vi "AnalyseNISTvsFlukeResults.vi"(8 "error in (no error)":errorcluster, 10 "AllData In":T4 {"FlukeData"."DataAnalysisArray"."TimeStamp" format="%^<%.3X\n%x>T"; "FlukeData"."ModelDataArray"."FREQUENCY" format="%#_6f"; "FlukeData"."ModelDataArray"."TimeStamp" format="%^<%.3X\n%x>T"; "FlukeData"."PMUDataArray"."FREQUENCY" format="%#_6f"; "FlukeData"."PMUDataArray"."TimeStamp" format="%^<%.3X\n%x>T"; "NISTData"."DataAnlysisArray"."TimeStamp" format="%^<%.3X\n%x>T"; "NISTData"."DUTDataArray"."Time Stamp" format="%^<%.3X\n%x>T"; "NISTData"."NIDataArray"."Time Stamp" format="%^<%.3X\n%x>T"}, 11 "NISTResults":T3 {"Time Stamp" format="%^<%.3X\n%x>T"}) -> (0 "error out":errorcluster, 3 "Resultarray":T1[](array[typedef]) {"Time Stamp" format="%^<%.3X\n%x>T"})   [LabVIEW 2014]
uses:
  typedefs/Alldata.ctl
  typedefs/NISTData.ctl
  typedefs/NIDataArray.ctl
  typedefs/NIData.ctl
  typedefs/PhasorRectangular.ctl
  typedefs/DUTData.ctl
  typedefs/NICalcAnalysis.ctl
  typedefs/CalcPhasorError.ctl
  typedefs/PlotDataArrays.ctl
  typedefs/PmuRawDataCluster.ctl
  typedefs/CalcAnalysis.ctl
  typedefs/ResultArray.ctl
  typedefs/Result.ctl
  typedefs/TVE_Fe_RFE.ctl
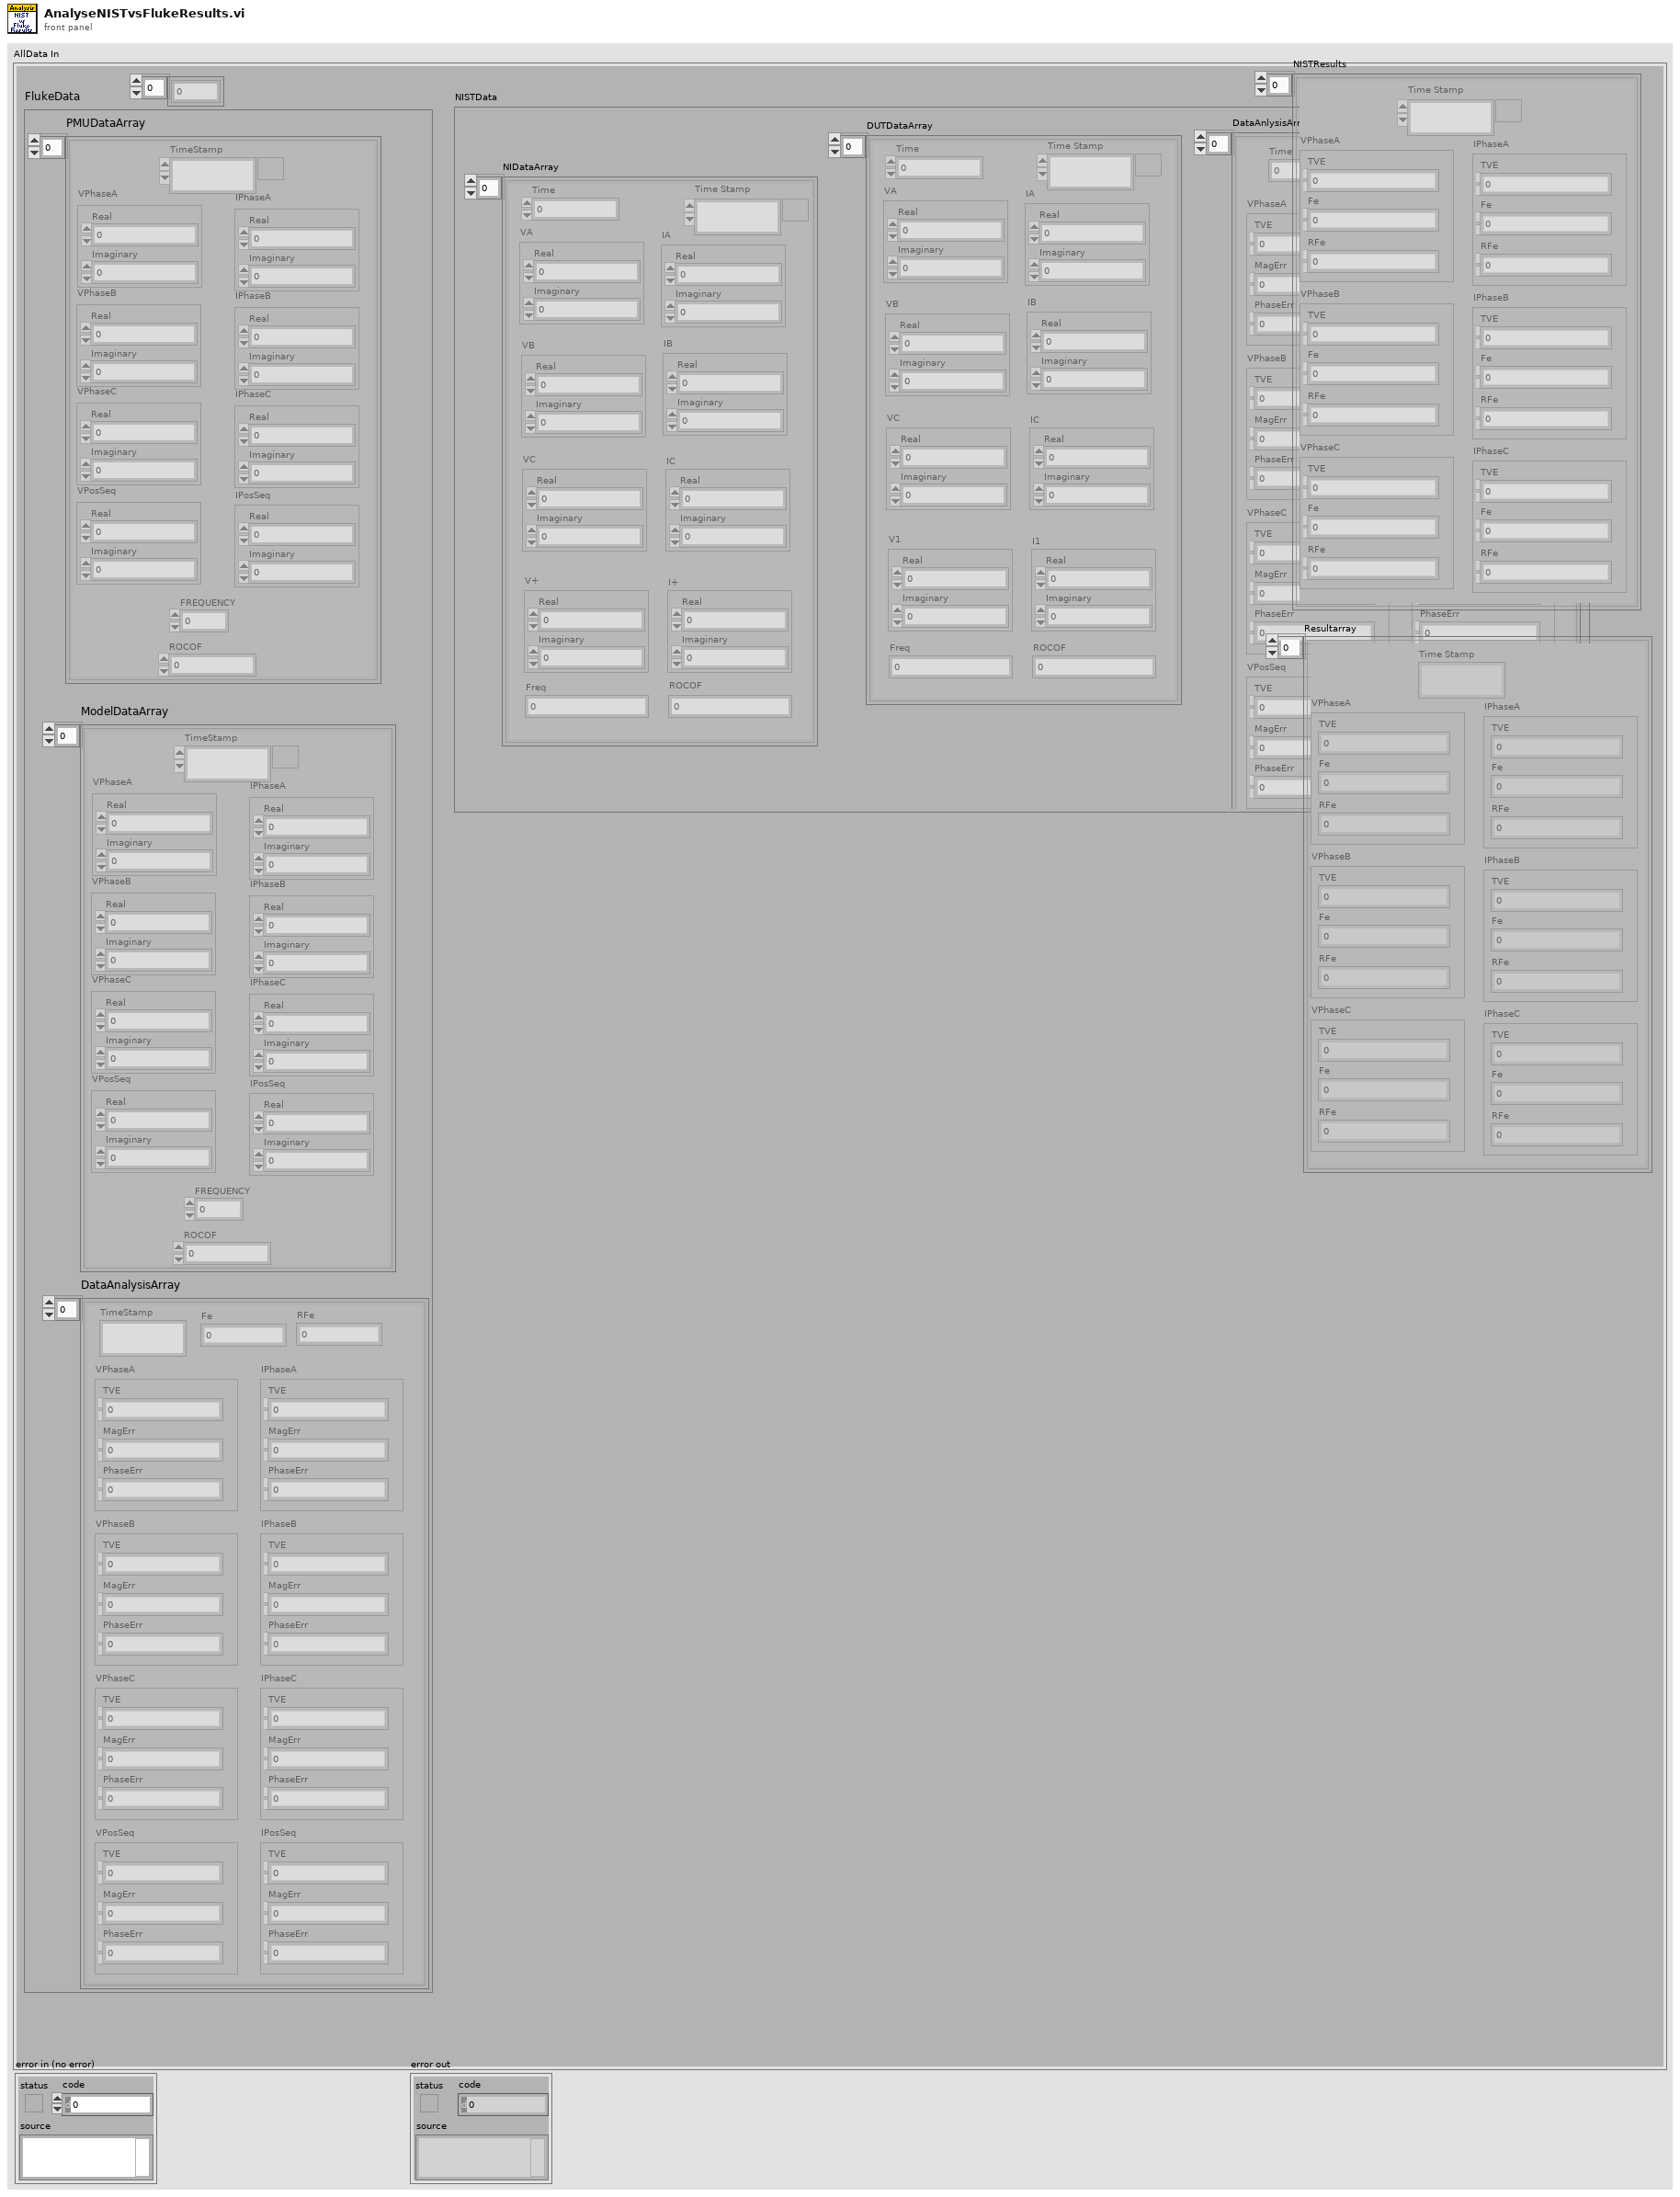
[diagram p1: front panel]
types:
  T1 = typedef "Result.ctl" = cluster{"Time Stamp":timestamp, "VPhaseA":T2, "VPhaseB":T2, "VPhaseC":T2, "IPhaseA":T2, "IPhaseB":T2, "IPhaseC":T2}
  T2 = typedef "TVE_Fe_RFE.ctl" = cluster{"TVE":dbl, "Fe":dbl, "RFe":dbl}
  T3 = typedef "ResultArray.ctl" = T1[]
  T4 = typedef "Alldata.ctl" = cluster{"NISTData":T5, "FlukeData":T12, "Params":dbl[]}
  T5 = typedef "NISTData.ctl" = cluster{"NIDataArray":T6, "DUTDataArray":T9[], "DataAnlysisArray":T10[]}
  T6 = typedef "NIDataArray.ctl" = T7[]
  T7 = typedef "NIData.ctl" = cluster{"Time":dbl, "VA":T8, "VB":T8, "VC":T8, "V+":T8, "IA":T8, "IB":T8, "IC":T8, "I+":T8, "Freq":dbl, "ROCOF":dbl, "Time Stamp":timestamp}
  T8 = typedef "PhasorRectangular.ctl" = cluster{"Real":dbl, "Imaginary":dbl}
  T9 = typedef "DUTData.ctl" = cluster{"Time":dbl, "VA":T8, "VB":T8, "VC":T8, "V1":T8, "IA":T8, "IB":T8, "IC":T8, "I1":T8, "Freq":dbl, "ROCOF":dbl, "Time Stamp":timestamp}
  T10 = typedef "NICalcAnalysis.ctl" = cluster{"Time":dbl, "VPhaseA":T11, "IPhaseA":T11, "VPhaseB":T11, "IPhaseB":T11, "VPhaseC":T11, "IPhaseC":T11, "VPosSeq":T11, "IPosSeq":T11, "Fe":dbl, "RFe":dbl, "TimeStamp":timestamp}
  T11 = typedef "CalcPhasorError.ctl" = cluster{"TVE":dbl, "MagErr":dbl, "PhaseErr":dbl}
  T12 = typedef "PlotDataArrays.ctl" = cluster{"PMUDataArray":T13[], "ModelDataArray":T13[], "DataAnalysisArray":T14[]}
  T13 = typedef "PmuRawDataCluster.ctl" = cluster{"TimeStamp":timestamp, "VPhaseA":T8, "VPhaseB":T8, "VPhaseC":T8, "VPosSeq":T8, "IPhaseA":T8, "IPhaseB":T8, "IPhaseC":T8, "IPosSeq":T8, "FREQUENCY":dbl, "ROCOF":sgl}
  T14 = typedef "CalcAnalysis.ctl" = cluster{"TimeStamp":timestamp, "VPhaseA":T11, "VPhaseB":T11, "VPhaseC":T11, "VPosSeq":T11, "IPhaseA":T11, "IPhaseB":T11, "IPhaseC":T11, "IPosSeq":T11, "Fe":dbl, "RFe":dbl}
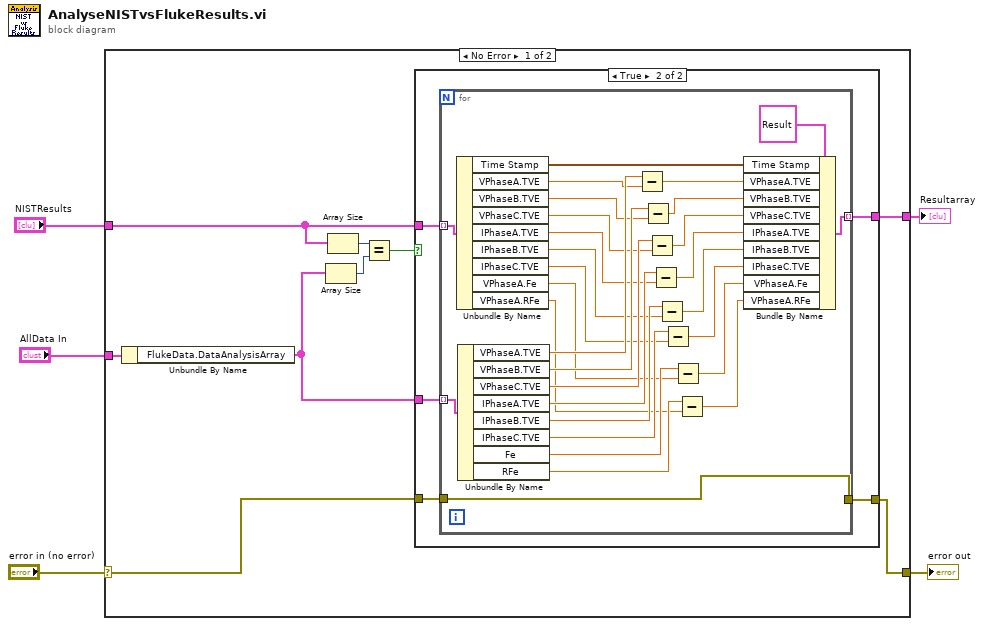
[diagram p0: block diagram]
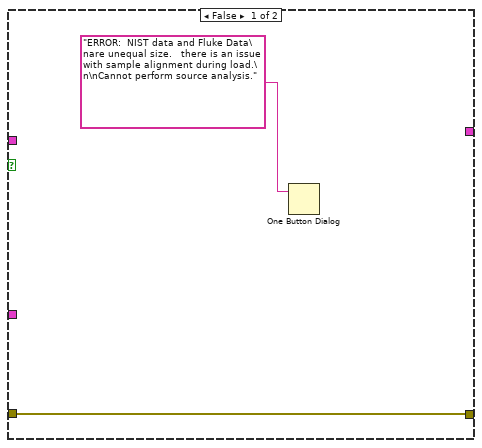
[diagram p2: hidden frame]
diagram:
  n1 = case shown="No Error" "error in (no error)" {
    selector: "error in (no error)" -> [w7 w52]
    tunnel: [w6 w52] -> w4
    tunnel: "AllData In" -> [w14 _]
    tunnel: "NISTResults" -> [w12 _]
    tunnel: [w8 _] -> w1
    frame No Error {
      n2 = Unbundle By Name(w14) -> ("FlukeData.DataAnalysisArray"=w11:T14[])
      n3 = Array Size(array=w11) -> (size(s)=w9:i32)
      n4 = Array Size(array=w12) -> (size(s)=w10:i32)
      n5 = Equal?(x=w10, y=w9) -> (x = y?=w13:bool)
      n6 = case shown="True" w13 {
        tunnel: w12 -> [_ w20]
        tunnel: w11 -> [_ w21]
        tunnel: [_ w19] -> w8
        tunnel: w7 -> [w16 w18]
        tunnel: [w16 w17] -> w6
        frame False {
          n7 = One Button Dialog(message="ERROR:  NIST data and Fluke Data\nare unequal size.   there is an issue with sample alignment during load.\n\nCannot perform source analysis.") -> ()  [unwired: 1 in, 1 out]
        }
        frame True {
          n8 = for {
            tunnel: w21 -> [w50] mode=indexing
            tunnel: w20 -> [w51] mode=indexing
            tunnel: [w41] -> w19 mode=indexing
            tunnel: w18 -> [w40]
            tunnel: [w40] -> w17
            n9 = Unbundle By Name(w51) -> ("Time Stamp"=w48:timestamp, "VPhaseA.TVE"=w38:dbl, "VPhaseB.TVE"=w36:dbl, "VPhaseC.TVE"=w34:dbl, "IPhaseA.TVE"=w32:dbl, "IPhaseB.TVE"=w30:dbl, "IPhaseC.TVE"=w28:dbl, "VPhaseA.Fe"=w25:dbl, "VPhaseA.RFe"=w24:dbl)
            n10 = Unbundle By Name(w50) -> ("VPhaseA.TVE"=w39:dbl, "VPhaseB.TVE"=w37:dbl, "VPhaseC.TVE"=w35:dbl, "IPhaseA.TVE"=w33:dbl, "IPhaseB.TVE"=w31:dbl, "IPhaseC.TVE"=w29:dbl, "Fe"=w27:dbl, "RFe"=w26:dbl)
            n11 = Subtract(x=w39, y=w38) -> (x-y=w47:dbl)
            n12 = Subtract(x=w37, y=w36) -> (x-y=w46:dbl)
            n13 = Subtract(x=w35, y=w34) -> (x-y=w45:dbl)
            n14 = Subtract(x=w33, y=w32) -> (x-y=w44:dbl)
            n15 = Subtract(x=w31, y=w30) -> (x-y=w43:dbl)
            n16 = Subtract(x=w29, y=w28) -> (x-y=w42:dbl)
            n17 = Subtract(x=w27, y=w25) -> (x-y=w23:dbl)
            n18 = Subtract(x=w26, y=w24) -> (x-y=w22:dbl)
            n19 = Bundle By Name(cluster=T1 {"Time Stamp"=timestamp(0 s since 1904-01-01), "VPhaseA"={"TVE"=0.0, "Fe"=0.0, "RFe"=0.0}, "VPhaseB"={"TVE"=0.0, "Fe"=0.0, "RFe"=0.0}, "VPhaseC"={"TVE"=0.0, "Fe"=0.0, "RFe"=0.0}, "IPhaseA"={"TVE"=0.0, "Fe"=0.0, "RFe"=0.0}, "IPhaseB"={"TVE"=0.0, "Fe"=0.0, "RFe"=0.0}, "IPhaseC"={"TVE"=0.0, "Fe"=0.0, "RFe"=0.0}} ("Result"), "Time Stamp"=w48, "VPhaseA.TVE"=w47, "VPhaseB.TVE"=w46, "VPhaseC.TVE"=w45, "IPhaseA.TVE"=w44, "IPhaseB.TVE"=w43, "IPhaseC.TVE"=w42, "VPhaseA.Fe"=w23, "VPhaseA.RFe"=w22) -> (w41:T1)
          }
        }
      }
    }
    frame Error {
    }
  }
  "error out" <- w4
  "Resultarray" <- w1
